vi "ChangePosition.vi"(8 "error in (no error)":errorcluster, 9 "Target value":dbl, 10 "Actual ref":refnum<vi>, 11 "Target ref":refnum<vi>) -> (0 "error out":errorcluster)   [LabVIEW 2013]
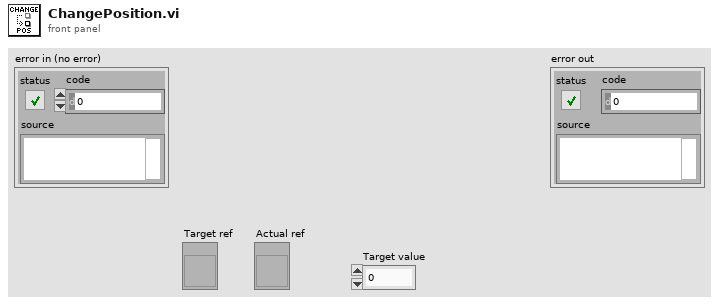
[diagram p1: front panel]
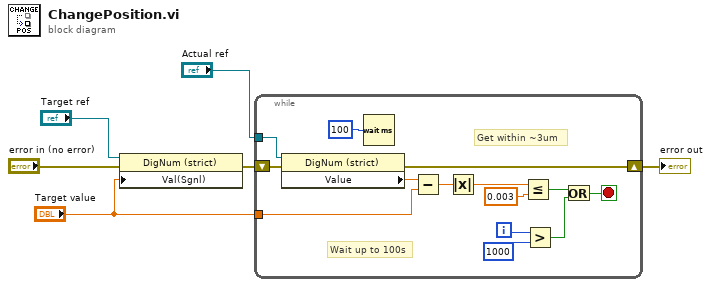
[diagram p0: block diagram]
diagram:
  n1 = property class="DigNum (strict)"(reference="Target ref", error in="error in (no error)", "Val(Sgnl)"="Target value") -> (error out=w4:errorcluster)  [unwired: 1 out]
  n2 = while {
    tunnel: "Target value" -> [w20]
    shift-right: [w13] -> w3
    shift-left: w4 -> [w14]
    tunnel: "Actual ref" -> [w12]
    i -> [w9]
    stop <- w11 stop-if-true
    # "Get within ~3um"
    # "Wait up to 100s"
    n3 = property class="DigNum (strict)"(reference=w12, error in=w14) -> (error out=w13:errorcluster, "Value"=w19:dbl)  [unwired: 1 out]
    n4 = Wait (ms)(milliseconds to wait=u32 100) -> ()  [unwired: 1 out]
    n5 = Subtract(x=w19, y=w20) -> (x-y=w18:dbl)
    n6 = Absolute Value(x=w18) -> (abs(x)=w17:dbl)
    n7 = Less Or Equal?(x=w17, y=0.003) -> (x <= y?=w10:bool)
    n8 = Greater?(x=w9, y=1000) -> (0:w7:bool)
    n9 = Or(x=w10, y=w7) -> (x .or. y?=w11:bool)
  }
  "error out" <- w3
